vi "Write Instrument.vi"(8 "error in (no error)":errorcluster, 10 "Instrument Driver":refnum<class "Instrument Driver.lvclass">, 11 "Instrument Sequencer in":refnum<class "Instrument Sequencer.lvclass">) -> (0 "error out":errorcluster, 3 "Instrument Sequencer out":refnum<class "Instrument Sequencer.lvclass">)   [LabVIEW 2020, in "Instrument Handler.lvlib" / "Instrument Sequencer.lvclass"]
doc: "Write the Instrument to the Instrument Sequencer."
uses:
  Instrument Sequencer.lvclass
  PPL/HDH.Actor Framework.Core.Instrument Driver.lvlibp/Instrument Driver/Instrument Driver.lvclass
  Instrument Sequencer.lvclass/Instrument Sequencer.ctl
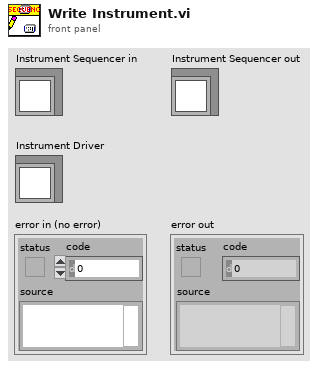
[diagram p1: front panel]
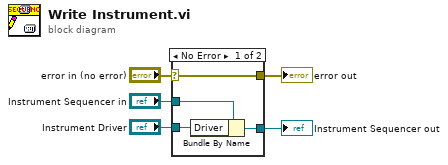
[diagram p0: block diagram]
diagram:
  n1 = case shown="No Error" "error in (no error)" {
    selector: "error in (no error)" -> [w9 w10]
    tunnel: [w9 w10] -> w4
    tunnel: [w7 w11] -> w2
    tunnel: "Instrument Sequencer in" -> [w8 w11]
    tunnel: "Instrument Driver" -> [w6 _]
    frame No Error {
      n2 = Bundle By Name(cluster=w8, "Driver"=w6) -> (w7:refnum<class "Instrument Sequencer.lvclass">)
    }
    frame Error {
    }
  }
  "error out" <- w4
  "Instrument Sequencer out" <- w2
